vi "PPG_Processing (SubVI).vi"(2 "Input PLETHY":dbl[](array[numeric]), 3 "Cycle NR":i32) -> (0 "LPF_ES":dbl[](array[numeric]), 1 "PSD":cluster{"f0":dbl, "df":dbl, "S(f)":dbl[]})   [LabVIEW 2015]
uses:
  <vilib>/Analysis/3filter.llb/Filter Passband Type.ctl
  <vilib>/Analysis/baseanly.llb/Scale 1D.vi
  <vilib>/Analysis/3filter.llb/FIR Filter (DBL).vi
  <vilib>/Analysis/2dsp.llb/Decimate (continuous, DBL).vi
  <vilib>/Analysis/NI_AALBase.lvlib
  <vilib>/Analysis/NI_AAL_SigProc.lvlib
  <vilib>/Analysis/NI_AALPro.lvlib
panel:
  out "error out":errorcluster
  in  "error in (no error)":errorcluster
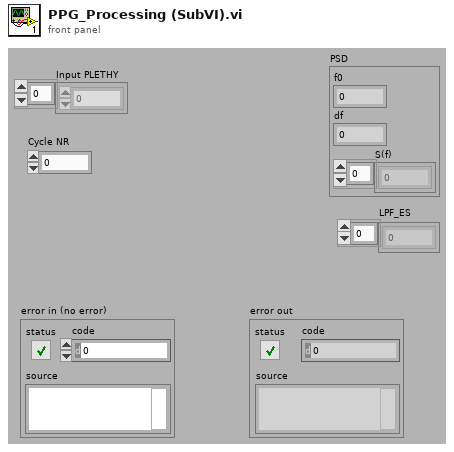
[diagram p1: front panel]
types:
  T1 = typedef "NI_AALBase.lvlib/Filter Passband Type.ctl" = enum32{"Lowpass", "Highpass", "Bandpass", "Bandstop"}
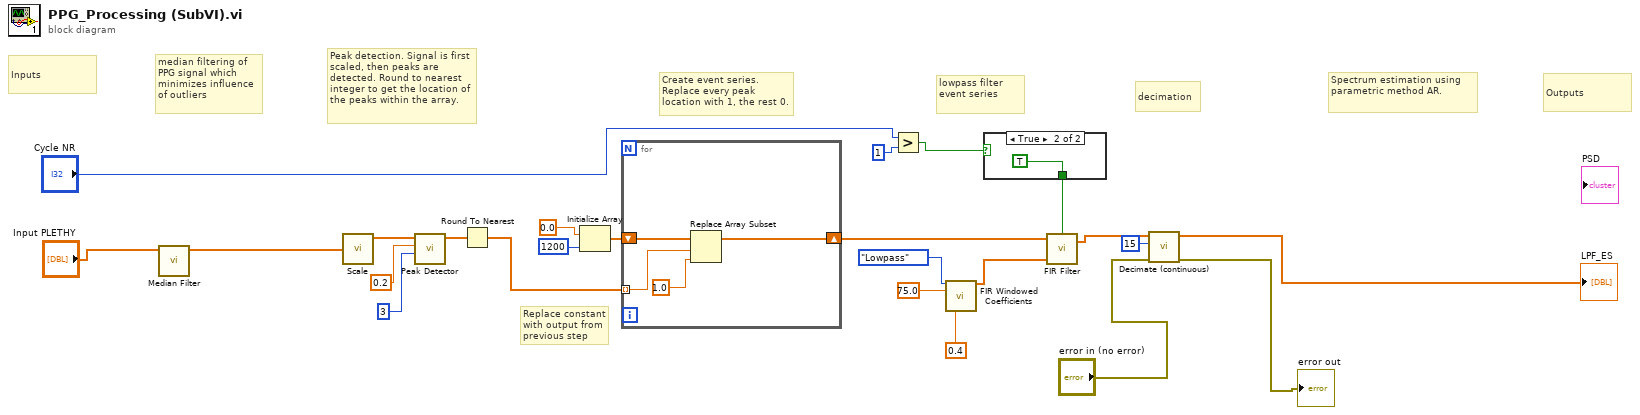
[diagram p0: block diagram]
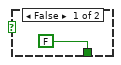
[diagram p2: hidden frame]
diagram:
  # "Outputs"
  # "Inputs"
  # "Replace constant with output from previous step"
  # "Create event series. Replace every peak location with 1, the rest 0."
  # "Spectrum estimation using parametric method AR."
  # "median filtering of PPG signal which minimizes influence of outliers"
  # "decimation"
  # "lowpass filter event series"
  # "Peak detection. Signal is first scaled, then peaks are detected. Round to nearest integer to get the location of the peaks within the array."
  n1 = call <vilib>:"Median Filter.vi"("X"="Input PLETHY") -> ("Filtered X"=w20:dbl[])  [unwired: 9 in, 1 out]
  n2 = call-poly <vilib>:"Scale.vi"("X"=w20) -> ("Y=(X-offset)/scale"=w19:dbl[])  [unwired: 3 out]
  n3 = call <vilib>:"Peak Detector.vi"("width"=3, "threshold"=0.2, "X"=w19) -> ("Locations"=w16:dbl[])  [unwired: 4 in, 4 out]
  n4 = Round To Nearest(number=w16) -> (nearest integer value=w15:dbl[])
  n5 = Initialize Array(0.0 ("element"), 1200 ("dimension size")) -> (w24:dbl[])
  n6 = for {
    shift-right: [w27] -> w14
    shift-left: w24 -> [w28]
    tunnel: w15 -> [w25] mode=indexing
    n7 = Replace Array Subset "Replace Array Subset"(array=w28, new element=1.0 ("new element/subarray"), index=w25) -> (w27:dbl[])
  }
  n8 = Greater?(x="Cycle NR", y=1) -> (0:w5:bool)
  n9 = call <vilib>:"FIR Windowed Coefficients.vi"("filter type"=Filter_Passband_Type."Lowpass", "sampling freq: fs"=75.0, "low cutoff freq: fl"=0.4) -> ("FIR Windowed Coefficients"=w13:dbl[])  [unwired: 11 in, 1 out]
  n10 = case shown="True" w5 {
    tunnel: [FALSE TRUE] -> w2
    frame False {
    }
    frame True {
    }
  }
  n11 = call-poly <vilib>:"FIR Filter.vi"("init/cont (init:F)"=w2, "FIR Coefficients"=w13, "X"=w14) -> ("Filtered X"=w9:dbl[])  [unwired: 1 in, 1 out]
  n12 = call-poly <vilib>:"Decimate (continuous).vi"("error in (no error)"="error in (no error)", "decimating factor"=15, "X"=w9) -> ("error out"=→"error out":errorcluster, "Decimated Array"=→"LPF_ES":dbl[])  [unwired: 7 in]
